vi "dispose_.vi"(8 "error in (no error)":errorcluster, 11 "Lua in":refnum<class "Lua.lvclass">) -> (0 "error out":errorcluster)   [LabVIEW 2020, in "Lua for LabVIEW.lvlib" / "Lua.lvclass"]
uses:
  Lua.lvclass
  private/lua_monitor_event.ctl
  Lua.lvclass/Lua.ctl
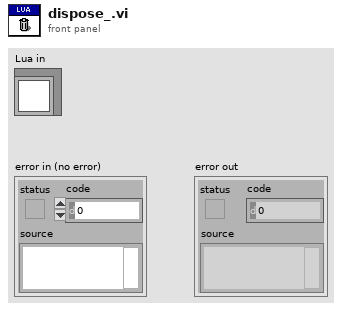
[diagram p1: front panel]
types:
  T1 = typedef "Lua for LabVIEW.lvlib/Lua.lvclass/lua_monitor_event.ctl" = enum16{"<null>", "terminate"}
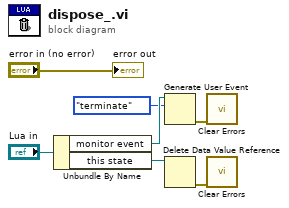
[diagram p0: block diagram]
diagram:
  n1 = Unbundle By Name("Lua in") -> ("monitor event"=w5:refnum<user-event>, "this state"=w3:refnum<data-value>)
  n2 = Generate User Event(user event=w5, event data cluster=lua_monitor_event."terminate" ("event data")) -> (error out=w2:errorcluster)  [unwired: 2 in, 1 out]
  n3 = Delete Data Value Reference(data value reference=w3) -> (error out=w1:errorcluster)  [unwired: 1 in, 1 out]
  n4 = call <vilib>:"Clear Errors.vi"("error in (no error)"=w2) -> ()  [unwired: 5 in, 2 out]
  n5 = call <vilib>:"Clear Errors.vi"("error in (no error)"=w1) -> ()  [unwired: 5 in, 2 out]
  "error out" <- "error in (no error)"
